vi "Bool2Number.vi"(1 "布尔":bool) -> (0 "数值":dbl)   [LabVIEW 2019]
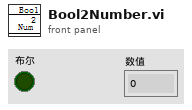
[diagram p1: front panel]
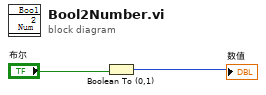
[diagram p0: block diagram]
diagram:
  n1 = Boolean To (0,1)(Boolean="布尔") -> (0, 1=→"数值":i16)
